vi "Device Init.vi"(0 "Device Port":refnum<visa-resource-name>, 5 "Baud Rate":u32=9600, 7 "Timeout":u32=10000, 9 "Bytes to Read":u32=52, 11 "Error In":errorcluster) -> (3 "Connected?":bool, 4 "VISA resource name":refnum<visa-resource-name>, 6 "Device":string, 8 "Serial Number":string, 15 "Error Out":errorcluster)   [LabVIEW 2025]
uses:
  a0c57d82-e86b-46b4-8ecc-c663b580368d.vi
  <vilib>/Instr/_visa.llb/VISA Configure Serial Port (Instr).vi
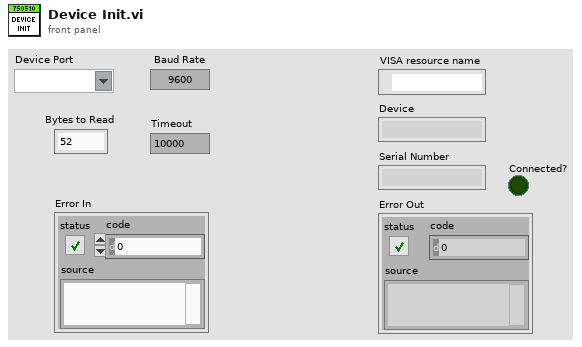
[diagram p1: front panel]
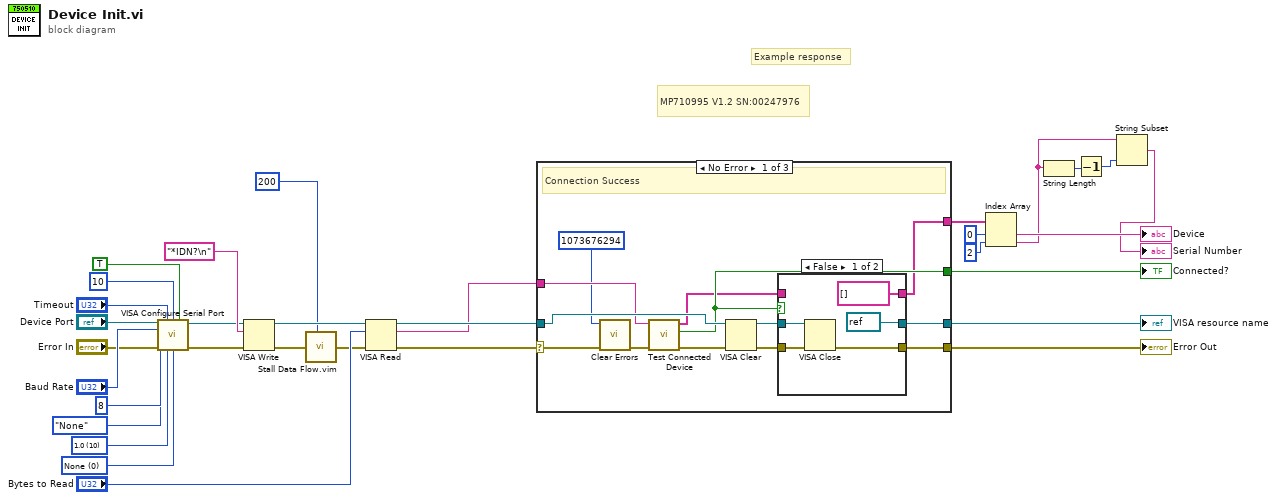
[diagram p0: block diagram]
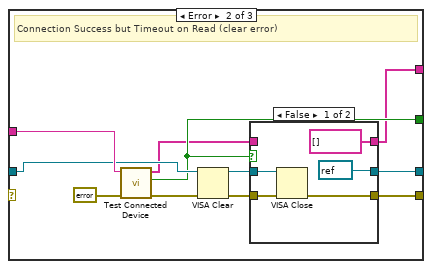
[diagram p3: hidden frame]
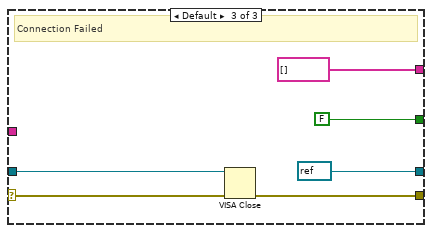
[diagram p5: hidden frame]
diagram:
  w16 = u16 10 items=["1.0"=10, "1.5"=15, "2.0"=20] ("Stop Bits")
  w15 = u16 0 items=["None", "XON/XOFF", "RTS/CTS", "XON/XOFF & RTS/CTS", "DTR/DSR", "XON/XOFF & DTR/DSR"] ("Flow Control")
  # "Example response"
  # "MP710995 V1.2 SN:00247976"
  n1 = call-poly "VISA Configure Serial Port"("VISA resource name"="Device Port", "timeout (10sec)"="Timeout", "termination char\n(0xA = '\\n' = LF)"=u8 10 ("Termination\nChar"), "Enable Termination\nChar (T)"=TRUE ("Enable Term\nChar"), "baud rate (9600)"="Baud Rate", "data bits (8)"=u16 8 ("Data Bits"), "parity (0:none)"=enum16{"None", "Odd", "Even", "Mark", "Space"}."None" ("Parity"), "error in (no error)"="Error In", "stop bits (10: 1 bit)"=w16, "flow control (0:none)"=w15) -> ("VISA resource name out"=w8:refnum<visa-resource-name>, "error out"=w9:errorcluster)  [unwired: 4 in]
  n2 = VISA Write(VISA resource name=w8, write buffer="*IDN?\n", error in (no error)=w9) -> (VISA resource name out=w31:refnum<visa-resource-name>, error out=w7:errorcluster)  [unwired: 1 out]
  n3 = call "Stall Data Flow.vim"("value in"=w7, "milliseconds to wait"=u32 200) -> ("value out"=w6:errorcluster)  [unwired: 1 out]
  n4 = VISA Read(VISA resource name=w31, byte count="Bytes to Read", error in (no error)=w6) -> (VISA resource name out=w28:refnum<visa-resource-name>, read buffer=w10:string, error out=w29:errorcluster)  [unwired: 1 out]
  n5 = case shown="No Error" w29 {
    selector: w29 -> [w38 _ w77]
    tunnel: w28 -> [w42 w63 w75]
    tunnel: w10 -> [w36 w64 _]
    tunnel: [w41 w59 w76] -> w26
    tunnel: [w40 w58 refnum<visa-resource-name> refnum ("VISA resource name")] -> w21
    tunnel: [w39 w62 FALSE] -> w27
    tunnel: [w33 w54 string[] [] ("Device Info")] -> w25
    frame No Error {
      # "Connection Success"
      n6 = call <vilib>:"Clear Errors.vi"("error in (no error)"=w38, "specific error code to clear (0: all)"=1073676294) -> ("error out"=w37:errorcluster)  [unwired: 4 in, 1 out]
      n7 = call "Test Connected Device.vi"("error in (no error)"=w37, "Read Buffer"=w36) -> ("error out"=w43:errorcluster, "Connected"=w39:bool, "Device Info"=w34:string[])  [unwired: 7 in]
      n8 = VISA Clear(VISA resource name=w42, error in (no error)=w43) -> (VISA resource name out=w44:refnum<visa-resource-name>, error out=w45:errorcluster)
      n9 = case shown="False" w39 {
        tunnel: [w50 w53] -> w41
        tunnel: w44 -> [w49 w52]
        tunnel: w45 -> [w48 w53]
        tunnel: [refnum<visa-resource-name> refnum ("VISA resource name") w52] -> w40
        tunnel: [string[] [] ("Device Info") w51] -> w33
        tunnel: w34 -> [_ w51]
        frame False {
          n10 = VISA Close(VISA resource name=w49, error in (no error)=w48) -> (error out=w50:errorcluster)
        }
        frame True {
        }
      }
    }
    frame Error {
      # "Connection Success but Timeout on Read (clear error)"
      n11 = call "Test Connected Device.vi"("error in (no error)"=errorcluster {"status"=FALSE, "code"=0, "source"=""} ("error IO"), "Read Buffer"=w64) -> ("error out"=w56:errorcluster, "Connected"=w62:bool, "Device Info"=w55:string[])  [unwired: 7 in]
      n12 = VISA Clear(VISA resource name=w63, error in (no error)=w56) -> (VISA resource name out=w60:refnum<visa-resource-name>, error out=w61:errorcluster)
      n13 = case shown="False" w62 {
        tunnel: [w69 w72] -> w59
        tunnel: w60 -> [w68 w71]
        tunnel: w61 -> [w67 w72]
        tunnel: [refnum<visa-resource-name> refnum ("VISA resource name") w71] -> w58
        tunnel: [string[] [] ("Device Info") w70] -> w54
        tunnel: w55 -> [_ w70]
        frame False {
          n14 = VISA Close(VISA resource name=w68, error in (no error)=w67) -> (error out=w69:errorcluster)
        }
        frame True {
        }
      }
    }
    frame Default {
      # "Connection Failed"
      n15 = VISA Close(VISA resource name=w75, error in (no error)=w77) -> (error out=w76:errorcluster)
    }
  }
  "Error Out" <- w26
  "Connected?" <- w27
  "VISA resource name" <- w21
  n16 = Index Array(array=w25, index #1=0 ("index"), index #2=2 ("index")) -> (element #1=→"Device":string, element #2=w2:string)
  n17 = String Length(string=w2) -> (length=w4:i32)
  n18 = Decrement(x=w4) -> (x-1=w3:i32)
  n19 = String Subset(string=w2, length (rest)=w3) -> (substring=→"Serial Number":string)  [unwired: 1 in]
